vi "CreateInMain.vi"(8 "error in (no error)":errorcluster, 10 "Broadcasts.Died":refnum<user-event>, 11 "JQMHModule in":refnum<class "RQMHModule.lvclass">) -> (0 "error out":errorcluster, 3 "JQMHModule out":refnum<class "RQMHModule.lvclass">, 5 "Event Registration Refnum":refnum<event-registration>)   [LabVIEW 2024, in "RQMHModule.lvclass"]
uses:
  RQMHModule.lvclass
  Shared/Died.ctl
  StandardRequests.ctl
  InitialiseArgs.ctl
  Reply.ctl
  StopEventArgs.ctl
  Show Front Panel--Args.ctl
  Hide Front Panel.ctl
  Show Block Diagram.ctl
  Hide Block Diagram--Args.ctl
  RQMHModule.lvclass/RQMHModule.ctl
  Shared/RQMHShared.lvlib
panel:
  out "Array":string[](array[string])
  out "call chain":string[](array[string])
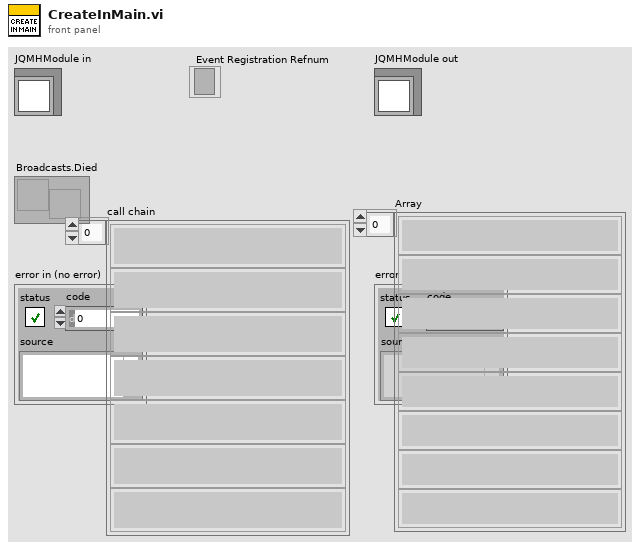
[diagram p1: front panel]
types:
  T1 = typedef "RQMHModule.lvclass/StandardRequests.ctl" = cluster{"Initialise":refnum<user-event>, "Stop Module":refnum<user-event>, "ShowFP":refnum<user-event>, "Hide Front Panel":refnum<user-event>, "Show Block Diagram":refnum<user-event>, "Hide Block Diagram":refnum<user-event>}
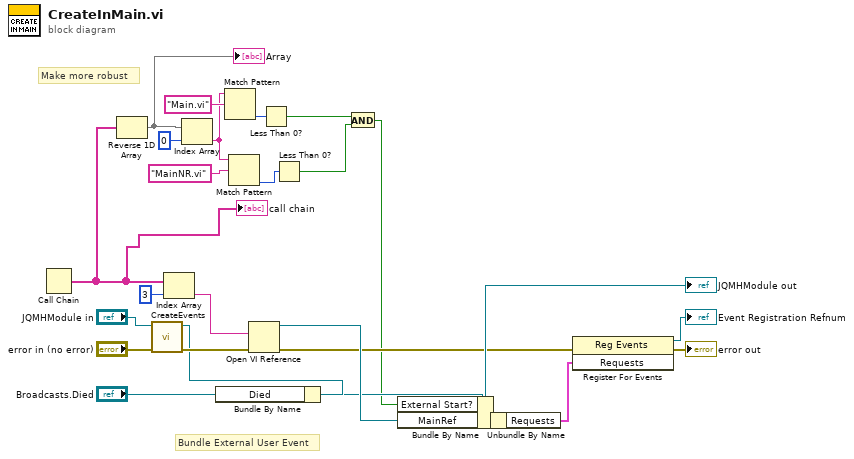
[diagram p0: block diagram]
diagram:
  # "Make more robust"
  # "Bundle External User Event"
  n1 = Call Chain() -> (call chain=w5:string[])
  "call chain" <- w5
  n2 = Reverse 1D Array(array=w5) -> (reversed array=w1:string[])
  "Array" <- w1
  n3 = call-dynamic "CreateEvents.vi"("error in (no error)"="error in (no error)", "JQMHCore in"="JQMHModule in") -> ("error out"=w21:errorcluster, "JQMHCore out"=w18:refnum<class "RQMHModule.lvclass">)  [unwired: 8 in]
  n4 = Index Array(array=w5, index=3) -> (element=w23:string)
  n5 = Index Array(array=w1, index=0) -> (element=w6:string)
  n6 = Bundle By Name(cluster=w18, "Died"="Broadcasts.Died") -> (w17:refnum<class "RQMHModule.lvclass">)
  n7 = Match Pattern(string=w6, regular expression="Main.vi") -> (offset past match=w9:i32)  [unwired: 1 in, 3 out]
  n8 = Match Pattern(string=w6, regular expression="MainNR.vi") -> (offset past match=w7:i32)  [unwired: 1 in, 3 out]
  n9 = Open VI Reference(vi path=w23, error in (no error)=w21) -> (vi reference=w22:refnum<vi>, error out=w13:errorcluster)  [unwired: 4 in]
  n10 = Less Than 0?(x=w9) -> (x < 0?=w4:bool)
  n11 = Less Than 0?(x=w7) -> (x < 0?=w3:bool)
  n12 = And(x=w4, y=w3) -> (x .and. y?=w2:bool)
  n13 = Bundle By Name(cluster=w17, "External Start?"=w2, "MainRef"=w22) -> (w16:refnum<class "RQMHModule.lvclass">)
  "JQMHModule out" <- w16
  n14 = Unbundle By Name(w16) -> ("Requests"=w15:T1)
  n15 = register-events(error in=w13, w15) -> (reference out=→"Event Registration Refnum":refnum<event-registration>, error out=→"error out":errorcluster)  [unwired: 1 in]
